vi "TCP-Simple-Server.vi"() -> ()   [LabVIEW 2019]
doc: "Demonstrates how to set up a basic TCP connection, send data to the specified port once a connection has been established, and terminate the connection once the data has been sent. This VI is designed to stop if the TCP connection is terminated. The data sent in this example is an array of random numbers."
panel:
  out "Chart":dbl[](graph)
  in  "Client Closed":string="The client VI closed the connection."
  in  "Stop":bool
  # "Overview: Demonstrates the use of the TCP functions to initialize a TCP server that can send data to a client VI.\nInstructions:\n1. Run the VI.\n2. Open TCP-Simple-Client.vi and follow the instructions on its- front panel. Note that if you wait longer than 30 seconds to do this after running this VI, it will time out.\n3. Click Stop to stop the VI. Note that if you stop the client VI, this VI will stop automatically."
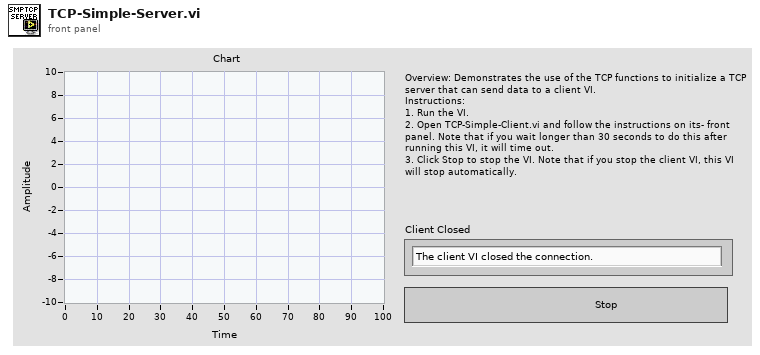
[diagram p1: front panel]
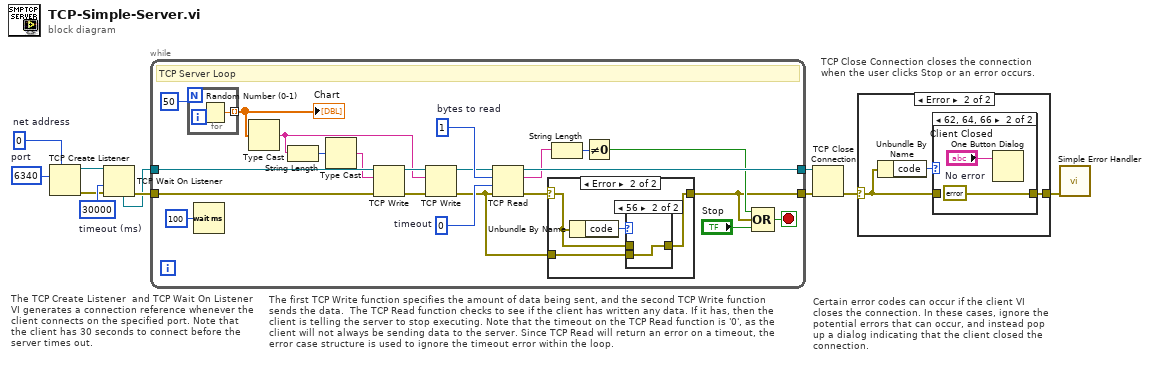
[diagram p0: block diagram]
diagram:
  w3 = u32 0  # net address
  w4 = u16 6340  # port
  w7 = 30000  # timeout (ms)
  # "TCP Close Connection closes the connection when the user clicks Stop or an error occurs."
  # "The TCP Create Listener  and TCP Wait On Listener VI generates a connection reference whenever the client connects on the specified port. Note that the client has 30 seconds to connect before the server times out."
  # "Certain error codes can occur if the client VI closes the connection. In these cases, ignore the potential errors that can occur, and instead pop up a dialog indicating that the client closed the connection."
  # "The first TCP Write function specifies the amount of data being sent, and the second TCP Write function sends the data.  The TCP Read function checks to see if the client has written any data. If it has, then the client is telling the server to stop executing. Note that the timeout on the TCP Read function is '0', as the client will not always be sending data to the server. Since TCP Read will return an error on a timeout, the error case structure is used to ignore the timeout error within the loop."
  n1 = TCP Create Listener(7:w3, 10:w4) -> (0:w2:errorcluster, 3:w1:refnum<k5>)  [unwired: 3 in, 1 out]
  n2 = TCP Wait On Listener(8:w2, 9:w7, 11:w1) -> (0:w6:errorcluster, 4:w5:refnum<k5>)  [unwired: 1 in, 3 out]
  n3 = while {
    tunnel: [w14] -> w10
    tunnel: [w20] -> w11
    tunnel: w5 -> [w33]
    tunnel: w6 -> [w24]
    stop <- w26 stop-if-true
    w19 = 0  # timeout
    w22 = 1  # bytes to read
    # "TCP Server Loop"
    n4 = for {
      N: 50 ("# of Points") -> [_]
      tunnel: [w41] -> w12 mode=indexing
      n5 = Random Number (0-1)() -> (number: 0 to 1=w41:dbl)
    }
    "Chart" <- w12
    n6 = Wait (ms)(milliseconds to wait=u32 100) -> ()  [unwired: 1 out]
    n7 = Type Cast(x=w12) -> (*(type *) &x=w28:string)  [unwired: 1 out]
    n8 = String Length(string=w28) -> (length=w30:i32)
    n9 = Type Cast(x=w30) -> (*(type *) &x=w29:string)  [unwired: 1 out]
    n10 = TCP Write(connection ID=w33, data in=w29, error in (no error)=w24) -> (connection ID out=w32:refnum<k5>, error out=w31:errorcluster)  [unwired: 2 out]
    n11 = TCP Write(connection ID=w32, data in=w28, error in (no error)=w31) -> (connection ID out=w21:refnum<k5>, error out=w13:errorcluster)  [unwired: 2 out]
    n12 = TCP Read(connection ID=w21, bytes to read=w22, error in (no error)=w13, 9:w19) -> (connection ID out=w20:refnum<k5>, data out=w17:string, error out=w15:errorcluster)  [unwired: 1 out]
    n13 = case shown="Error" w15 {
      selector: w15 -> [w34 w37]
      tunnel: [w34 w35] -> w14
      tunnel: w13 -> [_ w36]
      frame No Error {
      }
      frame Error {
        n14 = Unbundle By Name(w37) -> ("code"=w38:i32)
        n15 = case shown="56" w38 {
          tunnel: w37 -> [w39 _]
          tunnel: w36 -> [_ w40]
          tunnel: [w39 w40] -> w35
          frame Default {
          }
          frame 56 {
          }
        }
      }
    }
    n16 = String Length(string=w17) -> (length=w18:i32)
    n17 = Not Equal To 0?(x=w18) -> (x != 0?=w16:bool)
    n18 = Compound Arithmetic op=OR(w16, w14, "Stop") -> (w26:bool)
  }
  n19 = TCP Close Connection(connection ID=w11, error in (no error)=w10) -> (error out=w9:errorcluster)  [unwired: 2 out]
  n20 = case shown="Error" w9 {
    selector: w9 -> [w42 w44]
    tunnel: [w42 w43] -> w8
    frame No Error {
    }
    frame Error {
      n21 = Unbundle By Name(w44) -> ("code"=w45:i32)
      n22 = case shown="62, 64, 66" w45 {
        tunnel: w44 -> [w46 _]
        tunnel: [w46 w48] -> w43
        frame Default {
        }
        frame 62, 64, 66 {
          w48 = errorcluster {"status"=FALSE, "code"=0, "source"=""}  # No error
          n23 = One Button Dialog(message="Client Closed") -> ()  [unwired: 1 in, 1 out]
        }
      }
    }
  }
  n24 = call <vilib>:"Simple Error Handler.vi"("error in (no error)"=w8) -> ()  [unwired: 1 in, 8 out]
